vi "exnSpectralBlock spectral measurements power poly.vi"   [LabVIEW 2020]
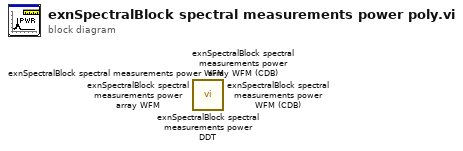
[diagram p0: block diagram]
diagram:
  n1 = call <vilib>:"exnSpectralBlock spectral measurements power DDT.vi"() -> ()  [unwired: 13 in, 3 out]
  n2 = call <vilib>:"exnSpectralBlock spectral measurements power array WFM (CDB).vi"() -> ()  [unwired: 13 in, 3 out]
  n3 = call <vilib>:"exnSpectralBlock spectral measurements power array WFM.vi"() -> ()  [unwired: 13 in, 3 out]
  n4 = call <vilib>:"exnSpectralBlock spectral measurements power WFM (CDB).vi"() -> ()  [unwired: 13 in, 3 out]
  n5 = call <vilib>:"exnSpectralBlock spectral measurements power WFM.vi"() -> ()  [unwired: 13 in, 3 out]
